vi "toNextSecond.vi"(7 "Values":i32[](array[numeric]), 11 "Cron in":T1) -> (3 "Cron out":T1)   [LabVIEW 2013, in "openCron.lvlib" / "Cron.lvclass"]
uses:
  Cron.lvclass
  CronTime -- cluster.ctl
  toNextHour.vi
  toNextDay.vi
  toNextMonth.vi
  <vilib>/LabVIEW Open Source Project/Epoch Date & Time/GregorianCal_MonthLength.vi
  updateWeekDay.vi
  toNextYear.vi
  <vilib>/LabVIEW Open Source Project/Epoch Date & Time/GregorianCal_MonthLengths.vi
  TimeStamp to Cron Time.vi
  Cron Time to TimeStamp.vi
  <vilib>/LabVIEW Open Source Project/Epoch Date & Time/isLeapYear (integer).vi
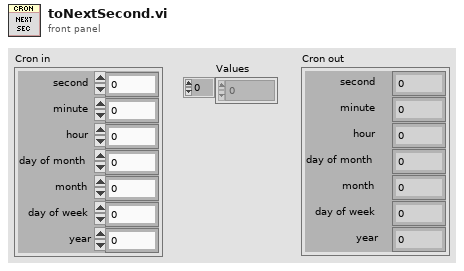
[diagram p1: front panel]
types:
  T1 = typedef "openCron.lvlib/Cron.lvclass/CronTime -- cluster.ctl" = cluster{"second":i32, "minute":i32, "hour":i32, "day of month":i32, "month":i32, "day of week":i32, "year":i32}
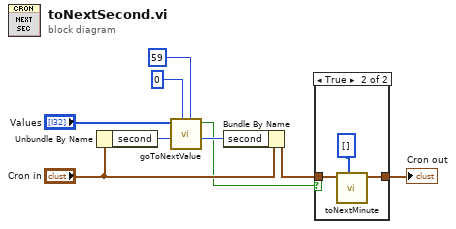
[diagram p0: block diagram]
diagram:
  n1 = Unbundle By Name("Cron in") -> ("second"=w4:i32)
  n2 = call "goToNextValue.vi"("maxValue"=59 ("upper limit"), "min Value"=0 ("lower limit"), "value in"=w4, "Values Pool"="Values") -> ("next value"=w3:i32, "RolledOver"=w2:bool)  [unwired: 6 in]
  n3 = Bundle By Name(cluster="Cron in", "second"=w3) -> (w8:T1)
  n4 = case shown="True" w2 {
    tunnel: w8 -> [w10 w13]
    tunnel: [w10 w12] -> w7
    frame False {
    }
    frame True {
      n5 = call "toNextMinute.vi"("Values"=i32[] [], "Cron in"=w13) -> ("Cron out"=w12:T1)  [unwired: 9 in]
    }
  }
  "Cron out" <- w7
